vi "GetHistory.vi"(8 "error in (no error)":errorcluster, 9 "Body":T1, 10 "OpState":variant, 11 "History":variant) -> (0 "error out":errorcluster, 2 "time series":T2)   [LabVIEW 2017, in "TestPanel.lvlib"]
uses:
  <vilib>/addons/InsightCM/Devices/Shared/Common/TestPanel/TestPanel.lvlib
  <vilib>/addons/InsightCM/MessageBus/Base/controls/TestPanelHistory.ctl
  <vilib>/addons/InsightCM/MessageBus/Base/controls/KeyValuePair.ctl
  <vilib>/addons/InsightCM/MessageBus/Base/controls/TestPanelTimeSeries.ctl
  <vilib>/addons/InsightCM/MessageBus/Base/controls/TestPanelValue.ctl
  <vilib>/addons/InsightCM/MessageBus/MessageLibrary/Device/controls/DeviceTestPanelGetTimeSeriesRequestBody.ctl
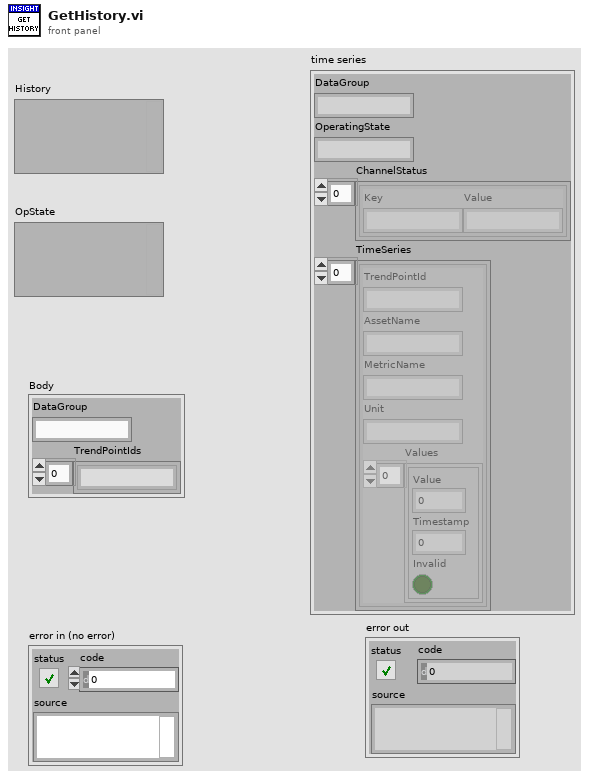
[diagram p1: front panel]
types:
  T1 = typedef "DeviceTestPanelGetTimeSeriesRequestBody.ctl" = cluster{"DataGroup":string, "TrendPointIds":string[]}
  T2 = typedef "TestPanelHistory.ctl" = cluster{"DataGroup":string, "OperatingState":string, "ChannelStatus":T3[], "TimeSeries":T4[]}
  T3 = typedef "KeyValuePair.ctl" = cluster{"Key":string, "Value":string}
  T4 = typedef "TestPanelTimeSeries.ctl" = cluster{"TrendPointId":string, "AssetName":string, "MetricName":string, "Unit":string, "Values":T5[]}
  T5 = typedef "TestPanelValue.ctl" = cluster{"Value":dbl, "Timestamp":i64, "Invalid":bool}
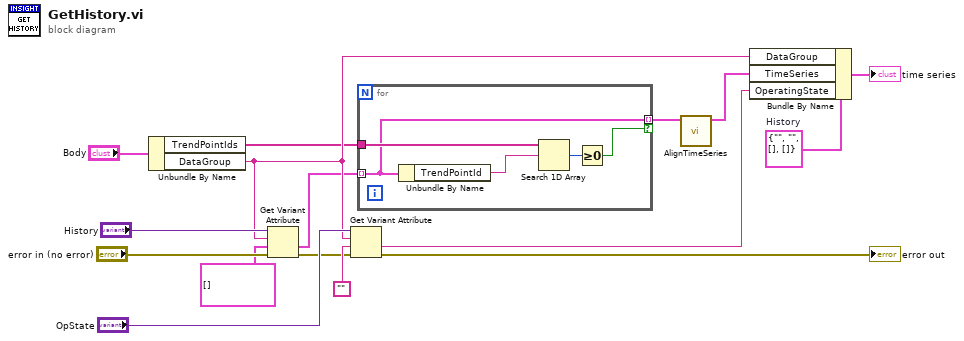
[diagram p0: block diagram]
diagram:
  w10 = T2 {"DataGroup"="", "OperatingState"="", "ChannelStatus"=[], "TimeSeries"=[]}  # History
  n1 = Unbundle By Name("Body") -> ("TrendPointIds"=w3:string[], "DataGroup"=w6:string)
  n2 = Get Variant Attribute(Variant="History", name=w6, default value (empty Variant)=T4[] [], error in="error in (no error)") -> (value=w4:T4[], error out=w7:errorcluster)  [unwired: 2 out]
  n3 = Get Variant Attribute(Variant="OpState", name=w6, default value (empty Variant)="", error in=w7) -> (value=w11:string, error out=→"error out":errorcluster)  [unwired: 2 out]
  n4 = for {
    tunnel: w4 -> [w18] mode=indexing
    tunnel: w3 -> [w21]
    tunnel: [w18] -> w1 mode=indexing if=w17
    n5 = Unbundle By Name(w18) -> ("TrendPointId"=w20:string)
    n6 = Search 1D Array(1D array=w21, element=w20) -> (index of element=w19:i32)  [unwired: 1 in]
    n7 = Greater Or Equal To 0?(x=w19) -> (x >= 0?=w17:bool)
  }
  n8 = call <vilib>:"AlignTimeSeries.vi"("time series in"=w1) -> ("time series out"=w2:T4[])  [unwired: 10 in]
  n9 = Bundle By Name(cluster=w10, "DataGroup"=w6, "TimeSeries"=w2, "OperatingState"=w11) -> (→"time series":T2)
